vi "SAPI Close Voice Object SubVI.vi"(8 "error in (no error)":errorcluster, 11 "speech object references":T1) -> (0 "error out":errorcluster)   [LabVIEW 2012, in "SAPI.TTS.lvlib"]
doc: "Closes the speech object references."
uses:
  SAPI.TTS.lvlib
  Controls/Speech object references.ctl
panel:
  # "Closes the speech object references."
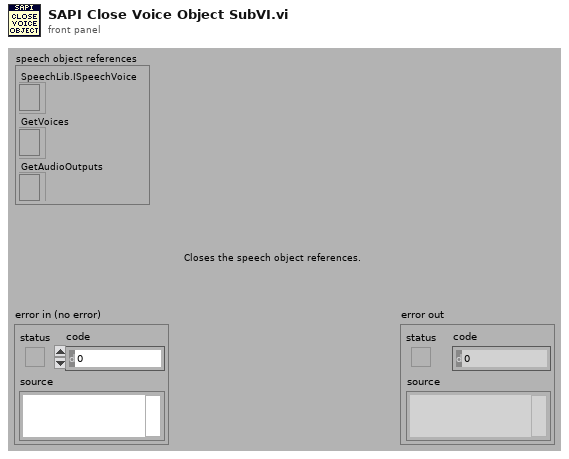
[diagram p1: front panel]
types:
  T1 = typedef "SAPI.TTS.lvlib/Speech object references.ctl" = cluster{"SpeechLib.ISpeechVoice":refnum<k7>, "GetVoices":refnum<k7>, "GetAudioOutputs":refnum<k7>}
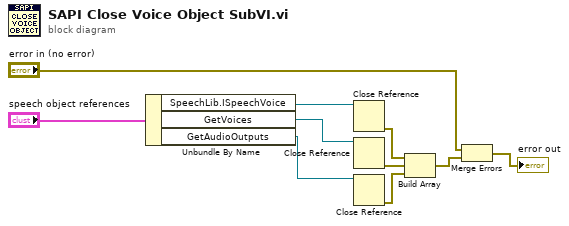
[diagram p0: block diagram]
diagram:
  n1 = Unbundle By Name("speech object references") -> ("SpeechLib.ISpeechVoice"=w9:refnum<k7>, "GetVoices"=w8:refnum<k7>, "GetAudioOutputs"=w7:refnum<k7>)
  n2 = Close Reference(reference=w9) -> (error out=w5:errorcluster)  [unwired: 1 in]
  n3 = Close Reference(reference=w8) -> (error out=w4:errorcluster)  [unwired: 1 in]
  n4 = Close Reference(reference=w7) -> (error out=w6:errorcluster)  [unwired: 1 in]
  n5 = Build Array(w5, w4, w6) -> (w3:errorcluster[])
  n6 = Merge Errors("error in (no error)", w3) -> (→"error out":errorcluster)
